vi "Get Position Size of Object.vi"(0 "Object Attributes":T1, 5 "Evaluate Pane Move":bool, 11 "error in (no error)":errorcluster, 12 "Force Hide":bool) -> (4 "Left":i32, 6 "Top":i32, 8 "Height":u32, 10 "Width":u32, 14 "Hidden":bool, 15 "error out":errorcluster)   [LabVIEW 2017, in "Front Panel Publisher.lvlib" / "Object.lvclass"]
doc: "This function will return the Left, Top, Height, and Width of a object passed in. This function will return all zeros if the object is not visible. This function also adjusts the offsets for the border in the HTML page."
uses:
  Object.lvclass
  Coordinates.ctl
  Enum - Pane Coordinate Method.ctl
  Attributes.ctl
  <vilib>/Utility/miscctls.llb/LVRectTypeDef.ctl
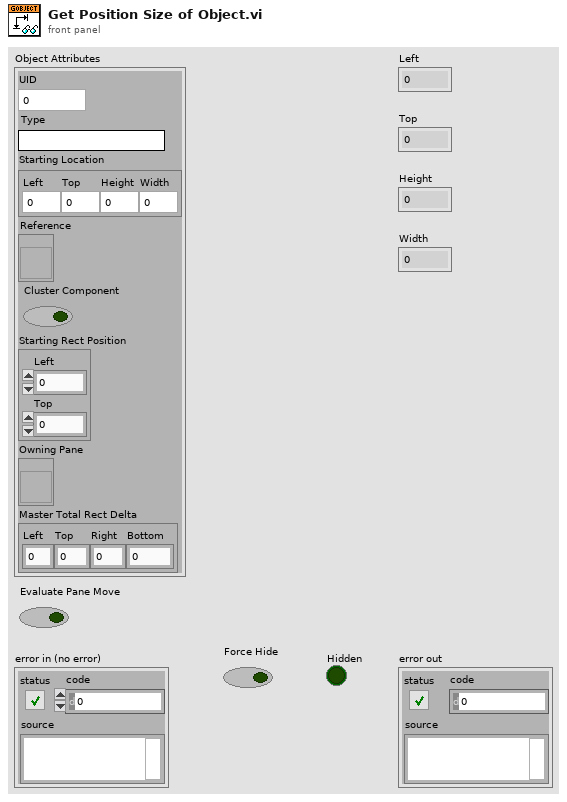
[diagram p1: front panel]
types:
  T1 = typedef "Front Panel Publisher.lvlib/Object.lvclass/Attributes.ctl" = cluster{"UID":i32, "Type":string, "Starting Location":T2, "Reference":refnum<vi>, "Cluster Component":bool, "Starting Rect Position":cluster{"Left":i16, "Top":i16}, "Owning Pane":refnum<vi>, "Master Total Rect Delta":T3}
  T2 = typedef "Front Panel Publisher.lvlib/Object.lvclass/Coordinates.ctl" = cluster{"Left":i32, "Top":i32, "Height":u32, "Width":u32}
  T3 = typedef "LVRectTypeDef.ctl" = cluster{"Left":i16, "Top":i16, "Right":i16, "Bottom":i16}
  T4 = typedef "Front Panel Publisher.lvlib/Object.lvclass/Enum - Pane Coordinate Method.ctl" = enum16{"Initialize", "Get Last Pane Offset", "Update Pane Position"}
  T5 = typedef "LVPointTypeDef.ctl" = cluster{"Horizontal":i16, "Vertical":i16}
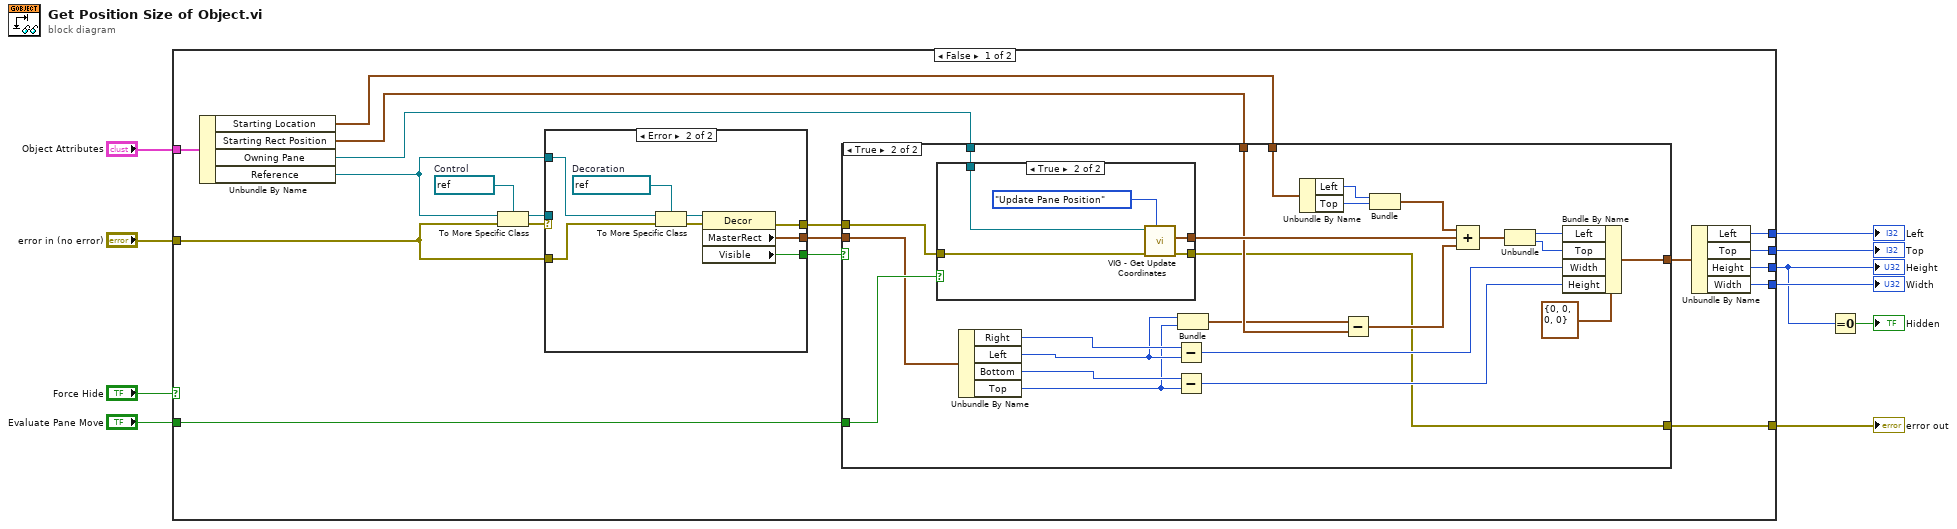
[diagram p0: block diagram]
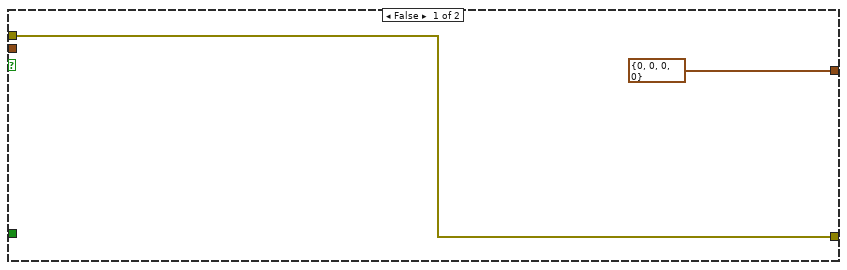
[diagram p2: hidden frame]
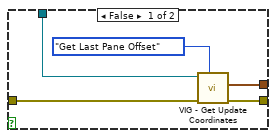
[diagram p3: hidden frame]
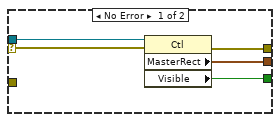
[diagram p4: hidden frame]
diagram:
  n1 = case shown="False" "Force Hide" {
    tunnel: [w29 _] -> w10
    tunnel: [w28 _] -> w2
    tunnel: [w11 w79] -> w9
    tunnel: [w25 _] -> w8
    tunnel: [w24 _] -> w7
    tunnel: "error in (no error)" -> [w19 w79]
    tunnel: "Evaluate Pane Move" -> [w18 _]
    tunnel: "Object Attributes" -> [w17 _]
    frame False {
      w23 = refnum<vi> refnum  # Control
      n2 = Unbundle By Name(w17) -> ("Starting Location"=w13:T2, "Starting Rect Position"=w12:cluster{"Left":i16, "Top":i16}, "Owning Pane"=w15:refnum<vi>, "Reference"=w16:refnum<vi>)
      n3 = To More Specific Class(target class=w23, reference=w16, error in=w19) -> (specific class reference=w22:refnum<vi>, error out=w27:errorcluster)
      n4 = case shown="Error" w27 {
        selector: w27 -> [w69 _]
        tunnel: [w70 w72] -> w14
        tunnel: [w68 w71] -> w26
        tunnel: w22 -> [w67 _]
        tunnel: [w66 w73] -> w20
        tunnel: w16 -> [_ w77]
        tunnel: w19 -> [_ w76]
        frame No Error {
          n5 = property class="Ctl"(reference=w67, error in=w69) -> (error out=w70:errorcluster, "MasterRect"=w66:T3, "Visible"=w68:bool)  [unwired: 1 out]
        }
        frame Error {
          w78 = refnum<vi> refnum  # Decoration
          n6 = To More Specific Class(target class=w78, reference=w77, error in=w76) -> (specific class reference=w75:refnum<vi>, error out=w74:errorcluster)
          n7 = property class="Decor"(reference=w75, error in=w74) -> (error out=w72:errorcluster, "MasterRect"=w73:T3, "Visible"=w71:bool)  [unwired: 1 out]
        }
      }
      n8 = case shown="True" w26 {
        tunnel: w20 -> [_ w42]
        tunnel: [T2 {"Left"=0, "Top"=0, "Height"=0, "Width"=0} ("Coordinates out") w33] -> w21
        tunnel: w18 -> [_ w54]
        tunnel: w15 -> [_ w55]
        tunnel: w14 -> [w30 w53]
        tunnel: w13 -> [_ w50]
        tunnel: w12 -> [_ w47]
        tunnel: [w30 w32] -> w11
        frame False {
        }
        frame True {
          n9 = case shown="True" w54 {
            tunnel: w55 -> [w56 w65]
            tunnel: [w57 w64] -> w48
            tunnel: w53 -> [w58 w63]
            tunnel: [w59 w62] -> w32
            frame False {
              n10 = call "VIG - Get Update Coordinates.vi"("Pane Method"=Enum_-_Pane_Coordinate_Method."Get Last Pane Offset", "error in (no error)"=w58, "Pane in"=w56) -> ("error out"=w59:errorcluster, "Offset From Start"=w57:T5)  [unwired: 6 in, 1 out]
            }
            frame True {
              n11 = call "VIG - Get Update Coordinates.vi"("Pane Method"=Enum_-_Pane_Coordinate_Method."Update Pane Position", "error in (no error)"=w63, "Pane in"=w65) -> ("error out"=w62:errorcluster, "Offset From Start"=w64:T5)  [unwired: 6 in, 1 out]
            }
          }
          n12 = Unbundle By Name(w42) -> ("Right"=w44:i16, "Left"=w41:i16, "Bottom"=w43:i16, "Top"=w40:i16)
          n13 = Subtract(x=w44, y=w41) -> (x-y=w38:i16)
          n14 = Subtract(x=w43, y=w40) -> (x-y=w37:i16)
          n15 = Bundle("Left"=w41, "Top"=w40) -> (w46:cluster{"Left":i16, "Top":i16})  [unwired: 1 in]
          n16 = Unbundle By Name(w50) -> ("Left"=w52:i32, "Top"=w51:i32)
          n17 = Subtract(x=w46, y=w47) -> (x-y=w45:cluster{"Left":i16, "Top":i16})
          n18 = Bundle("Left"=w52, "Top"=w51) -> (w49:cluster{"Left":i32, "Top":i32})  [unwired: 1 in]
          n19 = Compound Arithmetic op=ADD(w49, w48, w45) -> (w36:cluster{i32, i32})
          n20 = Unbundle(w36) -> (w35:i32, w34:i32)
          n21 = Bundle By Name(cluster=T2 {"Left"=0, "Top"=0, "Height"=0, "Width"=0} ("Coordinates in"), "Left"=w35, "Top"=w34, "Width"=w38, "Height"=w37) -> (w33:T2)
        }
      }
      n22 = Unbundle By Name(w21) -> ("Left"=w24:i32, "Top"=w25:i32, "Height"=w28:u32, "Width"=w29:u32)
    }
    frame True {
    }
  }
  "Width" <- w10
  "Height" <- w2
  "error out" <- w9
  "Top" <- w8
  "Left" <- w7
  n23 = Equal To 0?(x=w2) -> (x = 0?=→"Hidden":bool)
